vi "JSON to String Array.vi"(8 "error in (no error)":errorcluster, 10 "Parameter Name":string, 11 "JSON Tree In":variant) -> (0 "error out":errorcluster, 2 "Array":string[](array[string]), 3 "JSON Tree Out":variant)   [LabVIEW 2015, in "SLSC Switch.lvlib" / "SLSC Switch.lvclass"]
uses:
  SLSC Switch.lvclass
  <vilib>/LVH/i3 JSON/JSON Parsing/Get Object Parameter Files/Get Object Parameter - Array.vi
  <vilib>/LVH/i3 JSON/JSON Parsing/Get Array Value at Index Files/Get Array Value at Index - String.vi
  <vilib>/LVH/i3 JSON/i3-json.lvlib
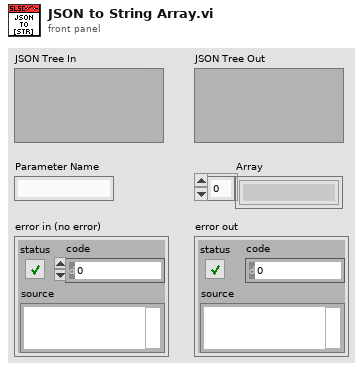
[diagram p1: front panel]
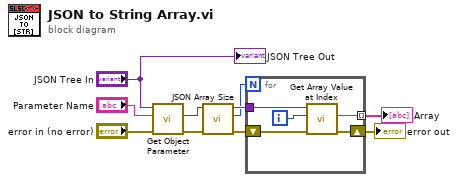
[diagram p0: block diagram]
diagram:
  n1 = call-poly <vilib>:"Get Object Parameter.vi"("error in (no error)"="error in (no error)", "Parameter Name"="Parameter Name", "JSON Tree In (JSON Object)"="JSON Tree In") -> ("error out"=w3:errorcluster, "JSON Array"=w7:variant)  [unwired: 5 in, 2 out]
  n2 = call <vilib>:"JSON Array Size.vi"("error in (no error)"=w3, "JSON Tree In (JSON Array)"=w7) -> ("error out"=w2:errorcluster, "Array Size"=w8:i32, "JSON Tree Passthrough (JSON Array)"=w9:variant)  [unwired: 7 in]
  n3 = for {
    N: w8 -> [_]
    tunnel: w9 -> [w15]
    tunnel: [w13] -> w10 mode=indexing
    shift-right: [w11] -> w1
    shift-left: w2 -> [w12]
    i -> [w14]
    n4 = call-poly <vilib>:"Get Array Value at Index.vi"("error in (no error)"=w12, "Index"=w14, "JSON Tree In (JSON Array)"=w15) -> ("error out"=w11:errorcluster, "String Value"=w13:string)  [unwired: 5 in, 2 out]
  }
  "Array" <- w10
  "error out" <- w1
  "JSON Tree Out" <- "JSON Tree In"
